vi "StartRamp.vi"(0 "handle in":i32, 1 "UnitAddress(0)":u16, 2 "MotNr(0)":u8, 5 "error in":errorcluster, 7 "TargetPosition(0)":i32) -> (14 "handle out":i32, 19 "error out":errorcluster)   [LabVIEW 2014, in "Sixpack - Driver.lvlib"]
doc: "ACHTUNG: Bei rotatorischen Achsen sind bei MT_NULLLEFT = 0 nur negative, bei MT_NULLLEFT = 1 nur positive Werte definiert! Der Motor fährt von der aktuellen Position auf die Zielposition. Das Kommando wird nicht ausgeführt, wenn der Motor noch in der Rampenfahrt ist. Um die Zielposition für einen sich bewegenden Motor zu ändern, siehe Kapitel 3.6.3\n\nCMD $23\nMotorNr (0...5)\nTargetPosition"
uses:
  Sixpack - Driver.lvlib
  DLL/PackDLL.dll
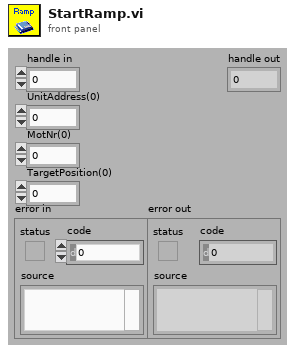
[diagram p1: front panel]
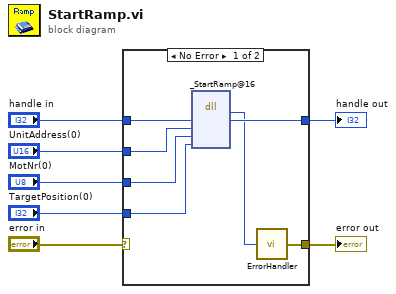
[diagram p0: block diagram]
diagram:
  n1 = case shown="No Error" "error in" {
    selector: "error in" -> [_ w15]
    tunnel: "handle in" -> [w14 w16]
    tunnel: [w13 w16] -> w6
    tunnel: "UnitAddress(0)" -> [w12 _]
    tunnel: "MotNr(0)" -> [w11 _]
    tunnel: "TargetPosition(0)" -> [w10 _]
    tunnel: [w8 w15] -> w2
    frame No Error {
      n2 = dll-call lib="D:/CS-Source/LV2014/GPL/instr.lib/SixPack/PackDLL/DLL/PackDLL.dll" fn="_StartRamp@16" label="StartRamp"("HANDLE"=w14, "UnitAddress"=w12, "MotNr"=w11, "TargetPosition"=w10) -> ("BOOLEAN"=w9:i8, "HANDLE"=w13:i32)  [unwired: 6 in, 2 out]
      n3 = call "ErrorHandler.vi"("BOOLEAN"=w9) -> ("error out"=w8:errorcluster)
    }
    frame Error {
    }
  }
  "handle out" <- w6
  "error out" <- w2
